vi "DBL to String (Async).vi"(11 "Format String":string="%.6f") -> (0 "error out":errorcluster, 2 "Promise out":refnum<class "Promise.lvclass">)   [LabVIEW 2020, in "Futures-Examples.lvlib"]
uses:
  Futures-Examples.lvlib
  Promises/Promise/Promise.lvclass
  DoubleValue/DoubleValue.lvclass
  StringValue/StringValue.lvclass
  DBL to String.vi
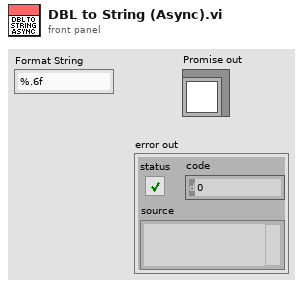
[diagram p1: front panel]
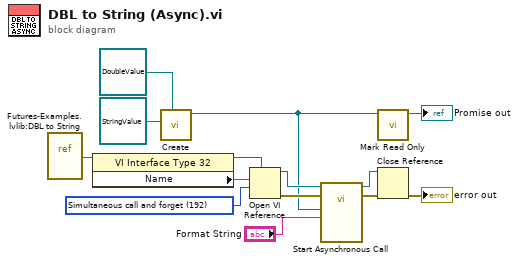
[diagram p0: block diagram]
diagram:
  w7 = 192 items=["Record modifications"=1, "Open templates for editing"=2, "Prompt user to save"=4, "Prepare for reentrant run"=8, "Prompt to find missing subVIs"=16, "Hide loading dialog box"=32, "Enable simultaneous calls"=64, "Prepare to call and forget"=128, "Simultaneous call and forget"=192, "Prepare to call and collect"=256, "Simultaneous call and collect"=320]
  n1 = vi-ref "Futures-Examples.lvlib:DBL to String.vi"() -> (w5:refnum<vi>)
  n2 = property class="VI Interface Type 32"(reference=w5) -> (reference out=w8:refnum<vi>, "Name"=w6:string)  [unwired: 1 in, 1 out]
  n3 = call "Create.vi"("Param Type (None)"=refnum<class "DoubleValue.lvclass"> refnum ("Futures-Examples.lvlib:DoubleValue.lvclass"), "Result Type"=refnum<class "StringValue.lvclass"> refnum ("Futures-Examples.lvlib:StringValue.lvclass")) -> ("Promise"=w4:refnum<class "Promise.lvclass">)  [unwired: 8 in, 1 out]
  n4 = Open VI Reference(type specifier VI Refnum (for type only)=w8, vi path=w6, options=w7) -> (vi reference=w10:refnum<vi>, error out=w9:errorcluster)  [unwired: 3 in]
  n5 = call-by-ref "Start Asynchronous Call"(reference=w10, error in=w9, "Format String"="Format String", "Promise"=w4) -> (reference out=w12:refnum<vi>, error out=w11:errorcluster)  [unwired: 10 in]
  n6 = call "Mark Read Only.vi"("Promise in"=w4) -> ("Promise out"=→"Promise out":refnum<class "Promise.lvclass">)  [unwired: 9 in, 1 out]
  n7 = Close Reference(reference=w12, error in (no error)=w11) -> (error out=→"error out":errorcluster)
